vi "APS get field bus a input plc.vi"(5 "RunStep":i16, 6 "AI_Value":dbl, 7 "Ch_No":i32, 8 "error in (no error)":errorcluster caption="错误输入（无错误）", 9 "MOD_No":i32, 10 "BUS_No":i32, 11 "Board_ID":i32) -> (0 "error out":errorcluster caption="错误输出", 3 "function return":i32, 4 "AI_Value out":dbl)   [LabVIEW 2011, in "APS168.lvlib"]
doc: "I32 FNTYPE APS_get_field_bus_a_input_plc( I32 Board_ID, I32 BUS_No, I32 MOD_No, I32 Ch_No, F64 *AI_Value, I16 RunStep );"
uses:
  APS168.lvlib
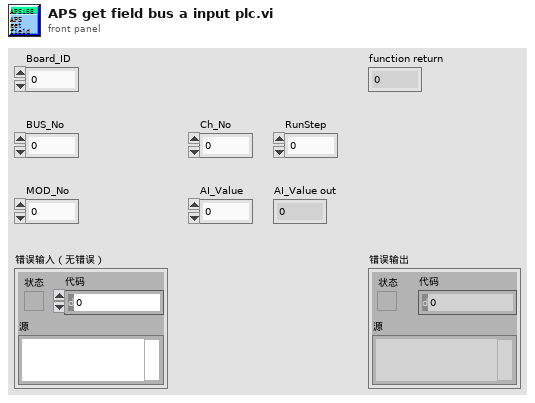
[diagram p1: front panel]
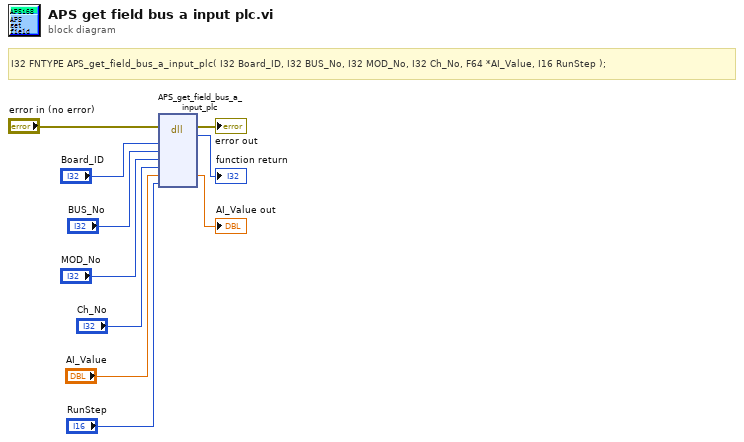
[diagram p0: block diagram]
diagram:
  # "I32 FNTYPE APS_get_field_bus_a_input_plc( I32 Board_ID, I32 BUS_No, I32 MOD_No, I32 Ch_No, F64 *AI_Value, I16 RunStep );"
  n1 = dll-call lib="PTH1Labs E软件ADLINK 204CAPS_1_7_1_LIB line 连续运动204APS168.*" fn="APS_get_field_bus_a_input_plc"(error in="error in (no error)", "Board_ID"="Board_ID", "BUS_No"="BUS_No", "MOD_No"="MOD_No", "Ch_No"="Ch_No", "AI_Value"="AI_Value", "RunStep"="RunStep") -> (error out=→"error out":errorcluster, →"function return":i32, "AI_Value"=→"AI_Value out":dbl)  [unwired: 7 in, 1 out]
